vi "labjack & attoDRY.vi"() -> (0 "error out":errorcluster)   [LabVIEW 2016]
uses:
  attoDRY - Drivers/APS - 100/Private/Element 8.ctl
  attoDRY - Drivers/attoDRY - Drivers.lvlib
panel:
  out "IMAG(千高斯)":dbl
  in  "电流磁场换算":dbl=1.2832
  in  "根据Trigger设置磁场":bool=TRUE
  in  "设置单位":enum16{"千高斯", "安培", ""}(ring)
  in  "毫秒倍数":u32=10
  out "单循环时间":u32(graph)
  in  "执行设置":bool
  out "error out 2":errorcluster
  in  "Sweep Control":cluster{T1, "Fast Sweep":bool, "是否暂停?":bool}
  in  "lower limit":dbl=-1.0 format="%.4f"
  in  "upper limit":dbl=1.0 format="%.4f"
  out "switch heater":bool
  out "lower sweep limit":dbl format="%.2f"
  out "upper sweep limit":dbl format="%.2f"
  out "Safety":T2
  out "Sweep State":T3
  out "Ausgangs-Cluster":T4
  in  "手动更新数据":bool
  in  "仅手动更新数据":bool=TRUE
  in  "VISA Resource Name":refnum<visa-resource-name>
  in  "ID Query (T: Check)":bool=TRUE
  in  "Reset (T: Reset)":bool=TRUE
  in  "Ring":u32(ring)=9600 items=["115200"=115200, "57600"=57600, "38400"=38400, "19200"=19200, "9600"=9600]
  out "trigger":bool
  in  "trigger level (V)":dbl
  in  "停止 2":bool
  in  "Negative Channel #":i32=199
  in  "quickSample":bool
  in  "longSettling":bool
  in  "Binary":bool
  in  "FirstFound":bool=TRUE
  in  "Address":string="1"
  out "Error Message":string
  out "模拟电压":dbl format="%.6f"
  in  "Positive Channel #":i32
  # "初始设置（运行前设置）"
  # "Error 信息"
  # "LabJack"
  # "attoDRY"
  # "千高斯/安培"
  # "Positive Channel 数字对应 LabJack 的AIN通道数字\nRing要与磁体控制箱上的波特率形同"
  # "LabJack 控制"
  # "attoDRY 状态"
  # "attoDRY 设置"
  # "程序控制"
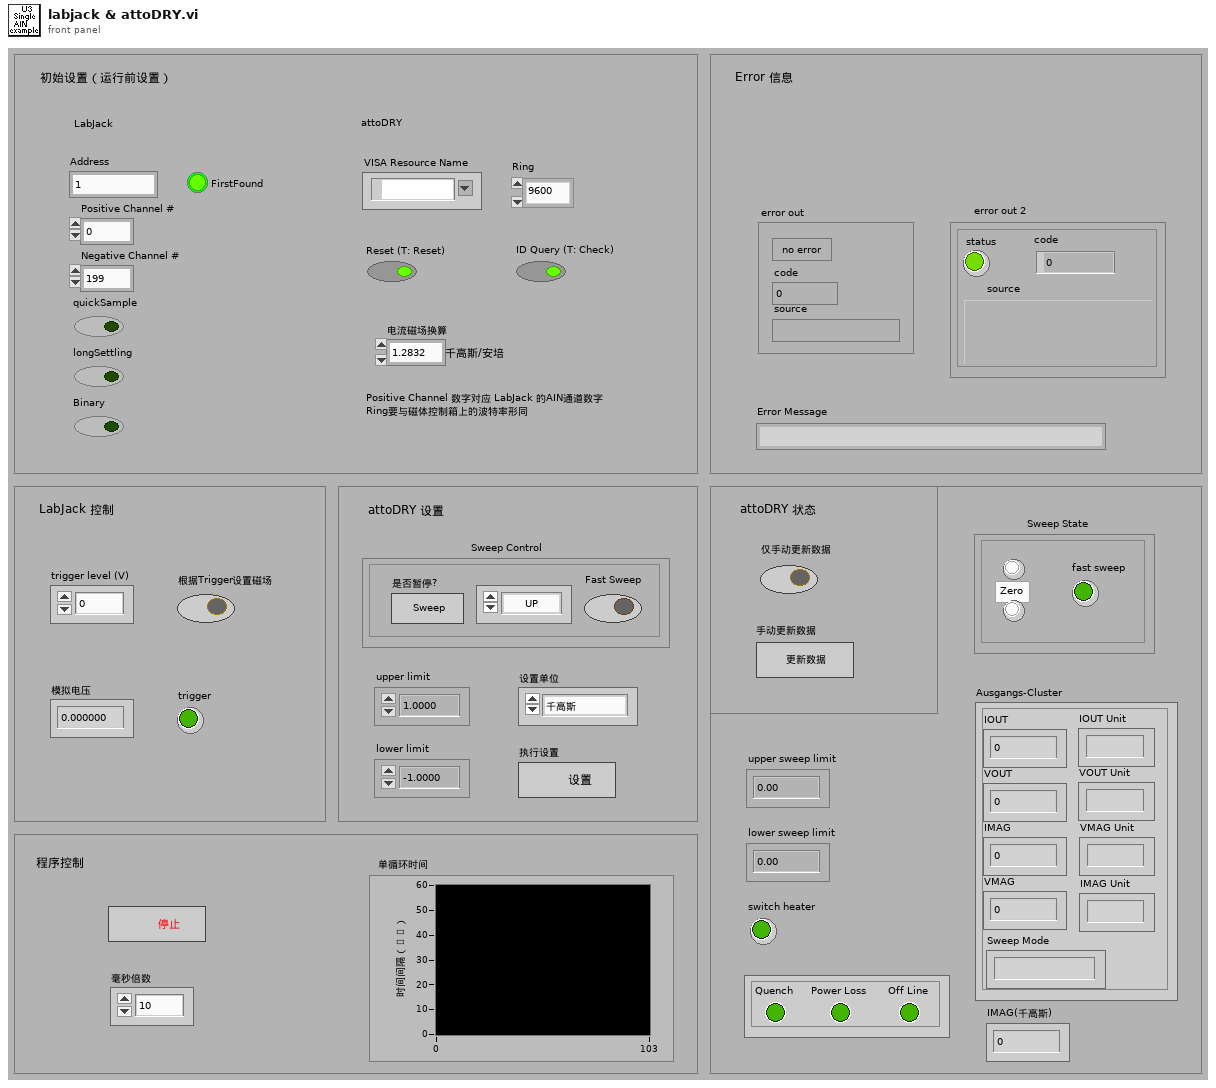
[diagram p1: front panel]
types:
  T1 = typedef "Element 8.ctl" = enum16{"UP", "to Zero", "Down"}
  T2 = cluster{"Power Loss":bool, "Off Line":bool, "Quench":bool}
  T3 = cluster{"zero":bool, "sweep down":bool, "sweep up":bool, "fast sweep":bool}
  T4 = cluster{"IOUT":dbl, "VOUT":dbl, "IMAG":dbl, "VMAG":dbl, "IOUT Unit":string, "VOUT Unit":string, "VMAG Unit":string, "IMAG Unit":string, "Sweep Mode":string}
  T5 = cluster{"Menüring":T1, "Fast Sweep":bool, "pause?":bool}
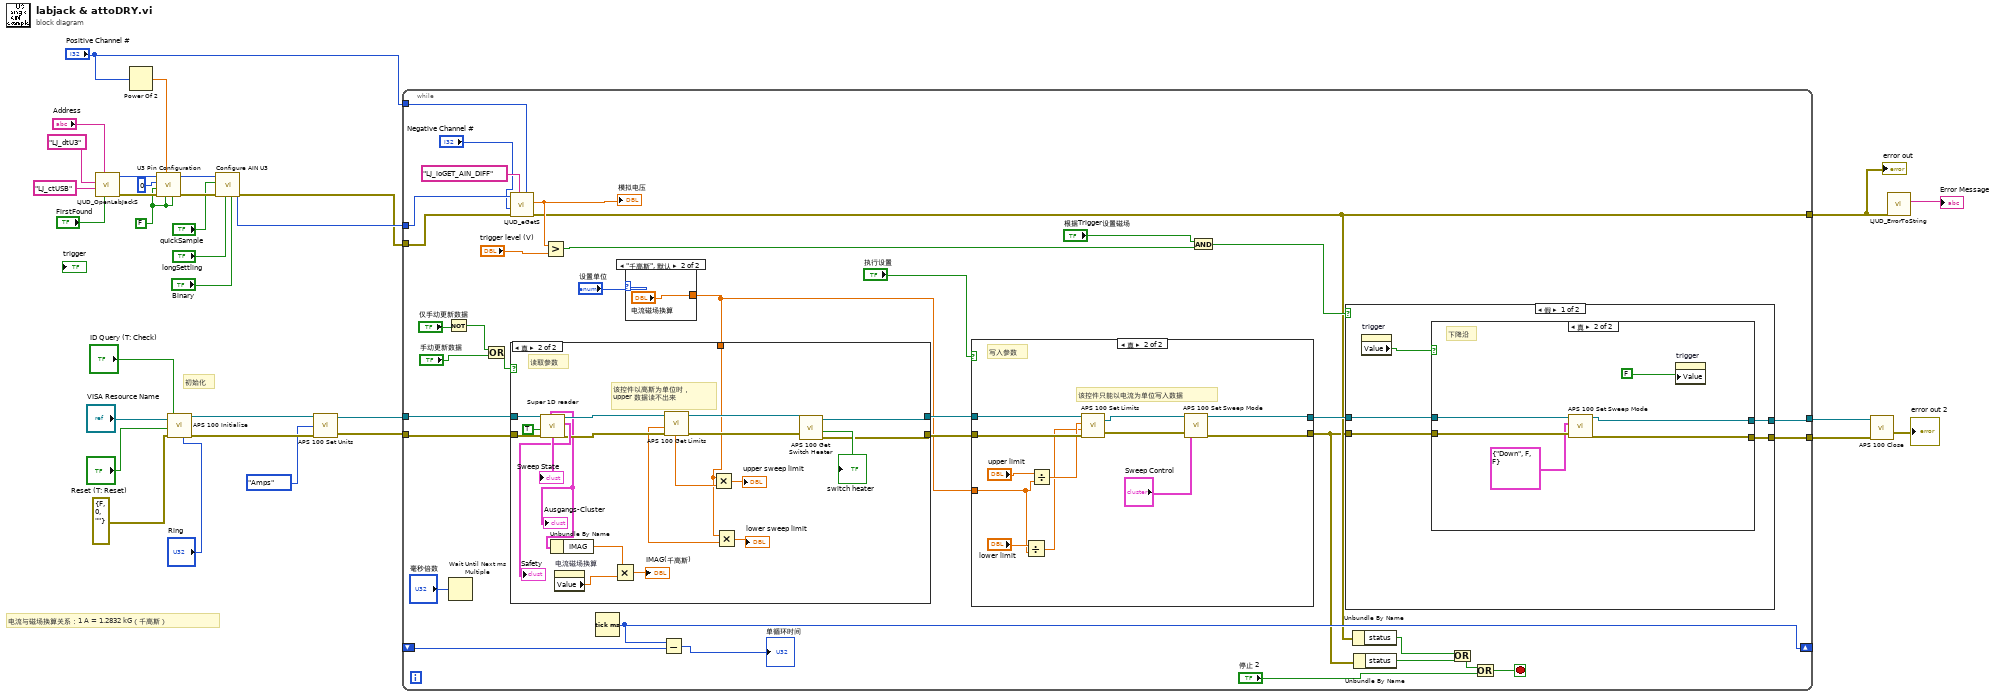
[diagram p0: block diagram]
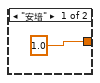
[diagram p2: hidden frame]
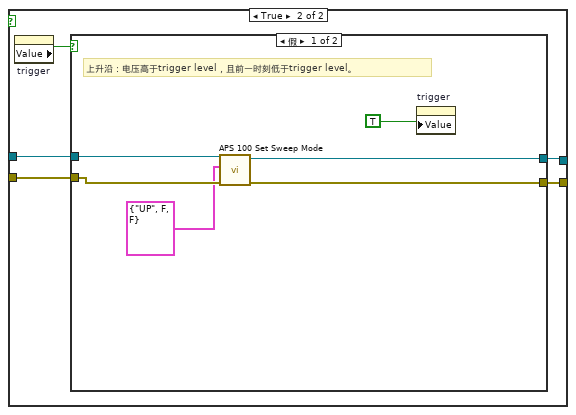
[diagram p6: hidden frame]
diagram:
  w20 = FALSE ("Enable DAC1")
  # "电流与磁场换算关系：1 A = 1.2832 kG（千高斯）"
  # "初始化"
  n1 = call "LJUD_OpenLabJackS.vi"("FirstFound"="FirstFound", "Address"="Address", "ConnectionType"="LJ_ctUSB", "DeviceType"="LJ_dtU3") -> ("error out"=w28:errorcluster, "Handle"=w26:i32)  [unwired: 5 in, 1 out]
  n2 = Power Of 2(x="Positive Channel #") -> (2^x=w22:dbl)
  n3 = call "U3 Pin Configuration.vi"("Enable Counter1"=w20, "Enable Counter0"=w20, "FIO/EIO Analog Enable"=w22, "error in"=w28, "Enable DAC1"=w20, "Number of Timers Enabled"=u8 0, "Handle In"=w26) -> ("error out"=w27:errorcluster, "Handle Out"=w25:i32)  [unwired: 3 in]
  n4 = call "APS 100 Initialize.vi"("VISA Resource Name"="VISA Resource Name", "ID Query (T: Check)"="ID Query (T: Check)", "Reset (T: Reset)"="Reset (T: Reset)", "error in (no error)"=errorcluster {"status"=FALSE, "code"=0, "source"=""}, "Ring"="Ring") -> ("VISA Resource Out"=w7:refnum<visa-resource-name>, "error out"=w6:errorcluster)  [unwired: 3 in]
  n5 = call "Configure AIN U3.vi"("Binary"="Binary", "longSettling"="longSettling", "error in"=w27, "quickSample"="quickSample", "Handle In"=w25) -> ("error out"=w16:errorcluster, "Handle Out"=w24:i32)  [unwired: 5 in]
  n6 = call "APS 100 Set Units.vi"("error in (no error)"=w6, "units"=enum16{"Amps", "Gauss"}."Amps", "VISA session"=w7) -> ("error out"=w4:errorcluster, "dup VISA session"=w5:refnum<visa-resource-name>)  [unwired: 1 in]
  n7 = while {
    tunnel: w24 -> [w66]
    tunnel: "Positive Channel #" -> [w65]
    tunnel: w16 -> [w63]
    tunnel: w5 -> [w56]
    tunnel: w4 -> [w55]
    tunnel: [w51] -> w9
    tunnel: [w50] -> w8
    shift-right: [w48] -> _
    shift-left: _ -> [w49]
    tunnel: [w36] -> w1
    stop <- w39 stop-if-true
    n8 = Not(x="仅手动更新数据") -> (.not. x?=w58:bool)
    n9 = Wait Until Next ms Multiple(millisecond multiple="毫秒倍数") -> ()  [unwired: 1 out]
    n10 = Or(x=w58, y="手动更新数据") -> (x .or. y?=w60:bool)
    n11 = call "LJUD_eGetS.vi"("Channel"=w65, "IOType"="LJ_ioGET_AIN_DIFF", "error in"=w63, "x1"="Negative Channel #", "Handle In"=w66) -> ("error out"=w36:errorcluster, "Value Read"=w62:dbl)  [unwired: 4 in, 1 out]
    "模拟电压" <- w62
    n12 = Greater?(x=w62, y="trigger level (V)") -> (0:w42:bool)
    n13 = Tick Count (ms)() -> (millisecond timer value=w48:u32)
    n14 = case shown="\"千高斯\", 默认" "设置单位" {
      tunnel: [1.0 "电流磁场换算"] -> w44
      frame "安培" {
      }
      frame "千高斯", Default {
      }
    }
    n15 = case shown="真" w60 {
      tunnel: w56 -> [w85 w106]
      tunnel: w55 -> [w84 w105]
      tunnel: [w85 w96] -> w54
      tunnel: [w84 w95] -> w53
      tunnel: w44 -> [_ w90]
      frame False {
      }
      frame True {
        # "该控件以高斯为单位时，\nupper 数据读不出来"
        # "读取参数"
        n16 = call "Super 1D reader.vi"("error in (no error)"=w105, "Persistant heater exists"=TRUE, "VISA session"=w106) -> ("error out 5"=w100:errorcluster, "Safety"=→"Safety":T2, "dup VISA session 4"=w101:refnum<visa-resource-name>, "Sweep Control"=→"Sweep State":T3, "Ausgangs-Cluster"=w89:T4)  [unwired: 3 in, 1 out]
        "Ausgangs-Cluster" <- w89
        n17 = Unbundle By Name(w89) -> ("IMAG"=w87:dbl)
        n18 = property on="电流磁场换算" class="DigNum (严格)"() -> ("Value"=w86:dbl)  [unwired: 2 in, 2 out]
        n19 = Multiply(x=w87, y=w86) -> (x*y=→"IMAG(千高斯)":dbl)
        n20 = call "APS 100 Get Limits.vi"("error in (no error)"=w100, "VISA session"=w101) -> ("error out"=w98:errorcluster, "lower sweep limit"=w91:dbl, "upper sweep limit"=w92:dbl, "dup VISA session"=w99:refnum<visa-resource-name>)  [unwired: 3 in, 1 out]
        n21 = Multiply(x=w90, y=w92) -> (x*y=→"upper sweep limit":dbl)
        n22 = Multiply(x=w90, y=w91) -> (x*y=→"lower sweep limit":dbl)
        n23 = call "APS 100 Get Switch Heater.vi"("VISA session"=w99, "error in (no error)"=w98) -> ("dup VISA session"=w96:refnum<visa-resource-name>, "switch heater"=→"switch heater":bool, "error out"=w95:errorcluster)  [unwired: 1 in]
      }
    }
    n24 = Subtract(x=w48, y=w49) -> (x-y=→"单循环时间":u32)
    n25 = case shown="真" "执行设置" {
      tunnel: w54 -> [w71 w83]
      tunnel: w53 -> [w70 w82]
      tunnel: [w71 w78] -> w52
      tunnel: [w70 w77] -> w35
      tunnel: w44 -> [_ w72]
      frame False {
      }
      frame True {
        # "该控件只能以电流为单位写入数据"
        # "写入参数"
        n26 = Divide(x="lower limit", y=w72) -> (x/y=w73:dbl)
        n27 = Divide(x="upper limit", y=w72) -> (x/y=w74:dbl)
        n28 = call "APS 100 Set Limits.vi"("VISA session"=w83, "upper limit"=w74, "lower limit"=w73, "error in (no error)"=w82) -> ("dup VISA session"=w81:refnum<visa-resource-name>, "error out"=w80:errorcluster)  [unwired: 1 in]
        n29 = call "APS 100 Set Sweep Mode.vi"("error in (no error)"=w80, "Sweep Control"="Sweep Control", "VISA session"=w81) -> ("error out"=w77:errorcluster, "dup VISA session"=w78:refnum<visa-resource-name>)  [unwired: 3 in]
      }
    }
    n30 = And(x="根据Trigger设置磁场", y=w42) -> (x .and. y?=w40:bool)
    n31 = case shown="假" w40 {
      tunnel: w52 -> [w110 w123]
      tunnel: w35 -> [w108 w122]
      tunnel: [w109 w121] -> w51
      tunnel: [w107 w120] -> w50
      frame False {
        n32 = property on="trigger" class="Bool (严格)"() -> ("Value"=w111:bool)  [unwired: 2 in, 2 out]
        n33 = case shown="真" w111 {
          tunnel: w110 -> [w113 w118]
          tunnel: [w113 w117] -> w109
          tunnel: w108 -> [w112 w116]
          tunnel: [w112 w115] -> w107
          frame False {
          }
          frame True {
            # "下降沿"
            n34 = call "APS 100 Set Sweep Mode.vi"("error in (no error)"=w116, "Sweep Control"=T5 {"Menüring"=enum."Down", "Fast Sweep"=FALSE, "pause?"=FALSE} ("Sweep Control 2"), "VISA session"=w118) -> ("error out"=w115:errorcluster, "dup VISA session"=w117:refnum<visa-resource-name>)  [unwired: 3 in]
            n35 = property on="trigger" class="Bool (严格)"("Value"=FALSE) -> ()  [unwired: 2 in, 2 out]
          }
        }
      }
      frame True {
        n36 = property on="trigger" class="Bool (严格)"() -> ("Value"=w124:bool)  [unwired: 2 in, 2 out]
        n37 = case shown="假" w124 {
          tunnel: w123 -> [w129 w132]
          tunnel: w122 -> [w128 w131]
          tunnel: [w126 w132] -> w121
          tunnel: [w125 w131] -> w120
          frame False {
            # "上升沿：电压高于trigger level，且前一时刻低于trigger level。"
            n38 = call "APS 100 Set Sweep Mode.vi"("error in (no error)"=w128, "Sweep Control"=T5 {"Menüring"=enum."UP", "Fast Sweep"=FALSE, "pause?"=FALSE} ("Sweep Control 2"), "VISA session"=w129) -> ("error out"=w125:errorcluster, "dup VISA session"=w126:refnum<visa-resource-name>)  [unwired: 3 in]
            n39 = property on="trigger" class="Bool (严格)"("Value"=TRUE) -> ()  [unwired: 2 in, 2 out]
          }
          frame True {
          }
        }
      }
    }
    n40 = Unbundle By Name(w36) -> ("status"=w34:bool)
    n41 = Unbundle By Name(w35) -> ("status"=w33:bool)
    n42 = Or(x=w34, y=w33) -> (x .or. y?=w37:bool)
    n43 = Or(x=w37, y="停止 2") -> (x .or. y?=w39:bool)
  }
  "error out" <- w1
  n44 = call "APS 100 Close.vi"("error in (no error)"=w8, "VISA session"=w9) -> ("error out"=→"error out 2":errorcluster)  [unwired: 9 in]
  n45 = call "LJUD_ErrorToString.vi"("error in"=w1) -> ("String"=→"Error Message":string)  [unwired: 10 in]
